vi "imp_test_v1_tmp.vi"() -> ()   [LabVIEW 2014]
uses:
  <vilib>/LabVIEW Targets/FPGA/cRIO/shared/nicrio_ModuleControls/nicrio_cRIO-9237_DataRatesRing.ctl
  <vilib>/LabVIEW Targets/FPGA/cRIO/shared/nicrio_ModuleControls/nicrio_cRIO-9237_ExcitationVoltageRing.ctl
  <vilib>/rvi/FXPMathLib/FxpSinAndCos/subVIs/nifxpmath_SinAndCos_SimConfig.ctl
  <vilib>/Platform/TimedLoop/XDataNode/timing_clust.ctl
  <vilib>/Platform/TimedLoop/XDataNode/nitl_modes.ctl
  <vilib>/Platform/TimedLoop/XDataNode/wakeup.ctl
  <vilib>/rvi/FXPMathLib/basic elements/FxpIntAccumulator/subVIs/nifxpmath_IntAccumulator_SimConfig.ctl
  <vilib>/rvi/FXPMathLib/FxpSqrt/subVIs/nifxpmath_Sqrt_SimConfig.ctl
  <vilib>/fxp/LVFixedPointOverflowPolicyTypeDef.ctl
  <vilib>/rvi/Emulation/niFpgaGetClockAttributes.vi
  <vilib>/rvi/Emulation/niFpgaSctlEmulationGetInTimedLoop.vi
  <vilib>/rvi/Emulation/niFpgaEmulationReportErrorSimple.vi
  <vilib>/rvi/Emulation/niFpgaProcessEmulError.vi
  <vilib>/rvi/interface/RandomDataEmulation/nirviRandomDataMultiElementFPGAFIFO.vi
  <instcachedir>/0/nirviRandomDataMultiElementFPGAFIFO_AD0CFC12EF974623A9C2E4184BC062B2.lvgen/nirviRandomDataMultiElementFPGAFIFO_AD0CFC12EF974623A9C2E4184BC062B2_023.vi
  <vilib>/rvi/interface/RandomDataEmulation/niFpgaRandomDataHandleErrors.vi
  <vilib>/rvi/Emulation/niFpgaCriticalErrorInLSC.vi
  <vilib>/rvi/eio/common/nirviEmuTemplateMethod_errors.vi
  <vilib>/rvi/FXPMathLib/FxpSinAndCos/simVIs/DllFxpSinAndCosTemp_sub.vi
  <vilib>/rvi/eio/common/nirviEmuTemplatePropertySet_errors.vi
  <vilib>/rvi/Analysis/common/codeGenErrors/XNode/niFpgaXNodeCodeGenErrorHandle.vi
  <vilib>/rvi/FXPMathLib/basic elements/FxpIntAccumulator/simVIs/DllFxpIntAccumulator_sub.vi
  <vilib>/rvi/FXPMathLib/FxpSqrt/simVIs/DllSqrtTemp_sub.vi
  <vilib>/rvi/DataTransferAndStorage/Container/XNode/niFpgaContainer.xnode
  <vilib>/rvi/interface/RandomDataEmulation/nirviRandomDataFpgaMultiElementTemplate.vi
  <vilib>/eio/EIONode/EIONode.xnode
  <vilib>/rvi/FXPMathLib/FxpMul/XNode/nifxpmath_Multiplier.xnode
  <vilib>/rvi/FXPMathLib/FxpSinAndCos/XNode/nifxpmath_SinAndCos.xnode
  <vilib>/rvi/Analysis/measure/butterworth/XNode/niFpgaButterworthFilter.xnode
  <vilib>/rvi/FXPMathLib/FxpSub/XNode/nifxpmath_Sub.xnode
  <vilib>/rvi/FXPMathLib/FxpAdd/XNode/nifxpmath_Add.xnode
  <vilib>/eio/EIOPropertyNode/EIOPropertyNode.xnode
  <vilib>/rvi/Analysis/measure/dc-rms/XNode/niFpgaDC-RMS.xnode
  <vilib>/Platform/TimedLoop/XDataNode/XDataNode.xnode
  <vilib>/rvi/FXPMathLib/basic elements/FxpIntAccumulator/XNode/nifxpmath_IntAccumulator.xnode
  <vilib>/rvi/FXPMathLib/FxpSqrt/XNode/nifxpmath_Sqrt.xnode
  <vilib>/rvi/eio/common/nirviEmuTemplatePropertyGet_errors.vi
  <vilib>/rvi/eio/common/nirviEmuTemplatePropertyGet_noerrors.vi
  <vilib>/rvi/eio/common/nirviEmuTemplatePropertySet_noerrors.vi
  <vilib>/Platform/TimedLoop/XDataNode/XDNodeRunTimeDep.lvlib
  <vilib>/rvi/FXPMathLib/sim/FxpSim.dll
panel:
  out "vb":fxp<+/-,38,8>
  out "va":fxp<+/-,38,8>
  out "ft_d2":fxp<+/-,64,59>
  out "Force_r":fxp<+/-,64,42>
  in  "Bv":fxp<+/-,22,8>
  out "D_error_dd":fxp<+/-,64,49>
  out "D_error_d":fxp<+/-,33,10>
  in  "Kv":fxp<+/-,22,8>
  out "D_error":fxp<+/-,64,33>
  out "Dr_sin_dd":fxp<+/-,64,48>
  out "Dr_sin_d":fxp<+/-,64,17>
  out "Sin omega":fxp<+/-,52,9>
  out "Dr_sin":fxp<+/-,39,10>
  in  "Sin offset":fxp<+/-,38,9>
  in  "Sin magnitude":fxp<+/-,22,7>
  out "Time now(s)":fxp<+,52,14>
  in  "Sin wave freq. (Hz)":fxp<+/-,32,6>
  in  "Dr":fxp<+/-,22,7>
  in  "Drive mode":i16(ring) items=["Backward", "Forward"]
  in  "F_d coeff.":i32[](array[numeric])=[946630756, 63555534]
  out "ft_d":fxp<+/-,36,25>
  out "D_dd":fxp<+/-,36,24>
  in  "D_dd coeff.":i32[](array[numeric])=[946630756, 63555534]
  out "dF_PID":fxp<+/-,36,33>
  in  "dF_PID coeff.":i32[](array[numeric])=[946630756, 63555534]
  out "ft_i":fxp<+/-,34,18>
  out "F_PID":fxp<+/-,51,14>
  in  "f_tolorance":fxp<+,22,6>
  in  "Ki":fxp<+/-,36,9>
  in  "Kd":fxp<+/-,36,9>
  out "f_tilde":fxp<+/-,33,11>
  in  "Kp":fxp<+/-,36,9>
  out "vq_F":fxp<+/-,20,5> format="%.57g"
  out "vd_F":fxp<+/-,20,5>
  in  "dF_add":bool
  out "D_d(mm/s)":fxp<+/-,41,10>
  out "omega(rad/s)":fxp<+/-,20,9>
  in  "Veolcity Estimation":i16(ring) items=["T method", "M_avg method", "M method"]
  in  "Stop motor":bool
  out "D_d(T)":fxp<+/-,41,10>
  out "omega(T)":fxp<+/-,20,9>
  in  "mt0_omega":u32
  out "mt_omega":u32
  out "rad(NrTheta)":fxp<+/-,33,10>
  out "D(mm)":fxp<+/-,32,10>
  out "Encoder Position":i32
  in  "Encoder reset":bool
  in  "Ini coe.":bool
  out "Loop rate (kHz)":fxp<+/-,36,7>
  out "Strain (RMS)":fxp<+,32,44>
  in  "Strain filter coeff.":i32[](array[numeric])=[-850883994, 1909449570, 3794062, -975456236, 2033039520, 4039635]
  out "Force":fxp<+/-,32,10>
  out "Strain":fxp<+/-,42,8>
  out "Fileterd data":fxp<+/-,32,4>
  out "Raw Force":fxp<+/-,32,10>
  in  "S/F coeff":fxp<+/-,41,4>
  out "Raw Strain":fxp<+/-,42,8>
  in  "Reset":bool
  in  "Stop (Strain)":bool
  out "Mod6/AI2":fxp<+/-,32,4>
  in  "Shunt Cal Enable":bool
  in  "Half-Bridge Enable":bool
  in  "Excitation Voltage":T1 items=["2.5 Volts", "3.3 Volts", "5.0 Volts", "10.0 Volts", "External Excitation"]
  in  "Data Rate":T2=1 items=["50.000 kS/s (NI 9237)"=1, "25.000 kS/s (NI 9237)"=2, "16.667 kS/s (NI 9237)"=3, "12.500 kS/s (NI 9237)"=4, "10.000 kS/s (NI 9237)"=5, "8.333 kS/s (NI 9237)"=6, "7.143 kS/s (NI 9237)"=7, "6.250 kS/s (NI 9237)"=8, "5.556 kS/s (NI 9237)"=9, "5.000 kS/s (NI 9237)"=10, "4.545 kS/s (NI 9237)"=11, "4.167 kS/s (NI 9237)"=12, "3.846 kS/s (NI 9237)"=13, "3.571 kS/s (NI 9237)"=14, "3.333 kS/s (NI 9237)"=15, "3.125 kS/s (NI 9237)"=16, "2.941 kS/s (NI 9237)"=17, "2.778 kS/s (NI 9237)"=18, "2.632 kS/s (NI 9237)"=19, "2.500 kS/s (NI 9237)"=20, "2.381 kS/s (NI 9237)"=21, "2.273 kS/s (NI 9237)"=22, "2.174 kS/s (NI 9237)"=23, "2.083 kS/s (NI 9237)"=24, "2.000 kS/s (NI 9237)"=25, "1.923 kS/s (NI 9237)"=26, "1.852 kS/s (NI 9237)"=27, "1.786 kS/s (NI 9237)"=28, "1.724 kS/s (NI 9237)"=29, "1.667 kS/s (NI 9237)"=30, "1.613 kS/s (NI 9237)"=31]
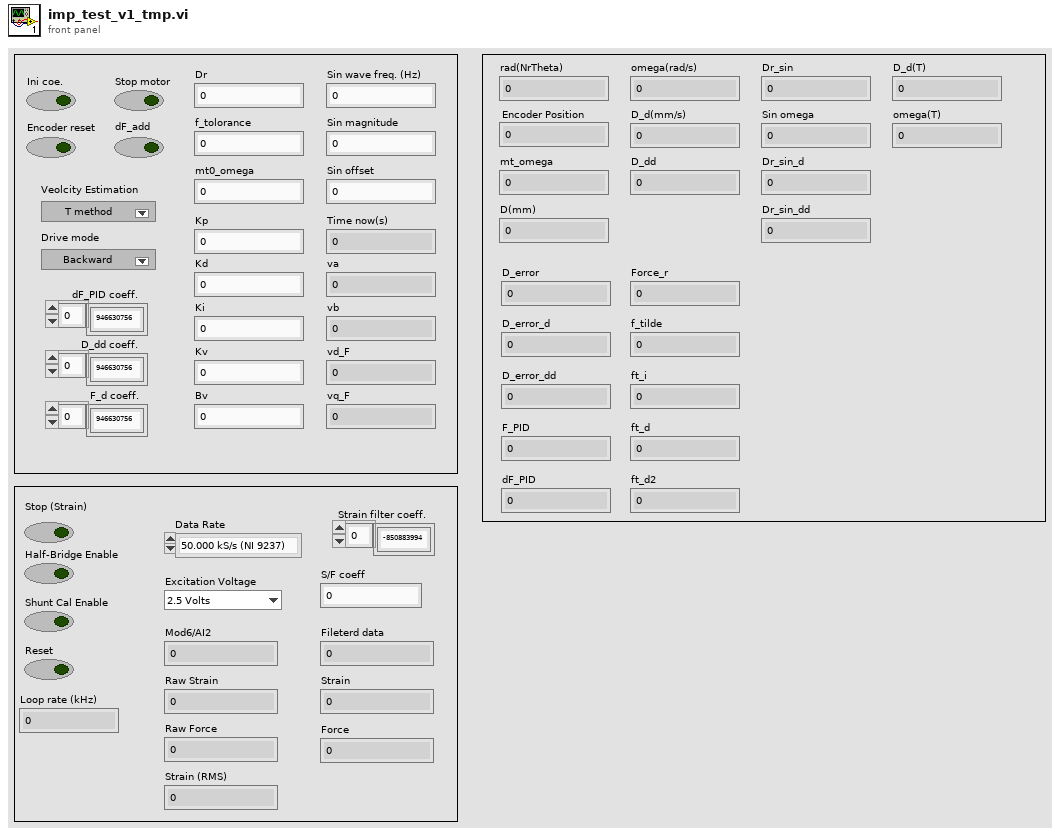
[diagram p1: front panel]
types:
  T1 = typedef "nicrio_cRIO-9237_ExcitationVoltageRing.ctl" = u8
  T2 = typedef "nicrio_cRIO-9237_DataRatesRing.ctl" = u8
  T3 = typedef "XDNodeRunTimeDep.lvlib/timing_clust.ctl" = cluster{"Expected End [f-1]":u64, "Actual End [f-1]":u64, "Finished Late? [f-1]":bool, "Expected End [i-1]":u64, "Actual End [i-1]":u64, "Finished Late? [i-1]":bool, "Expected Start [i]":u64, "Actual Start [i]":u64, "Expected Start [f]":u64, "Actual Start [f]":u64, "Source Name":string, "Structure Name":string, "Period":i64, "Deadline":i64, "Offset":i64, "Start":i64, "Priority":i32, "Timeout":i32, "Mode":T4, "Wakeup Reason":T5, "Error":errorcluster, "Source Type":string, "Secondary Source Type":string, "Global End Time":u64, "Global Start Time":u64, "Frame Duration":u64, "Iteration Duration":u64, "Assigned CPU":i32, "I/O Scan Engine Mode":u32}
  T4 = typedef "XDNodeRunTimeDep.lvlib/nitl_modes.ctl" = enum32{"No Change", "Process missed periods, maintain original phase", "Discard missed periods, maintain original phase", "Process missed periods, ignore original phase", "Discard missed periods, ignore original phase"}
  T5 = typedef "XDNodeRunTimeDep.lvlib/wakeup.ctl" = enum32{"Normal", "Aborted", "Asynchronous wakeup", "Timing source error", "Timed loop error", "Timeout"}
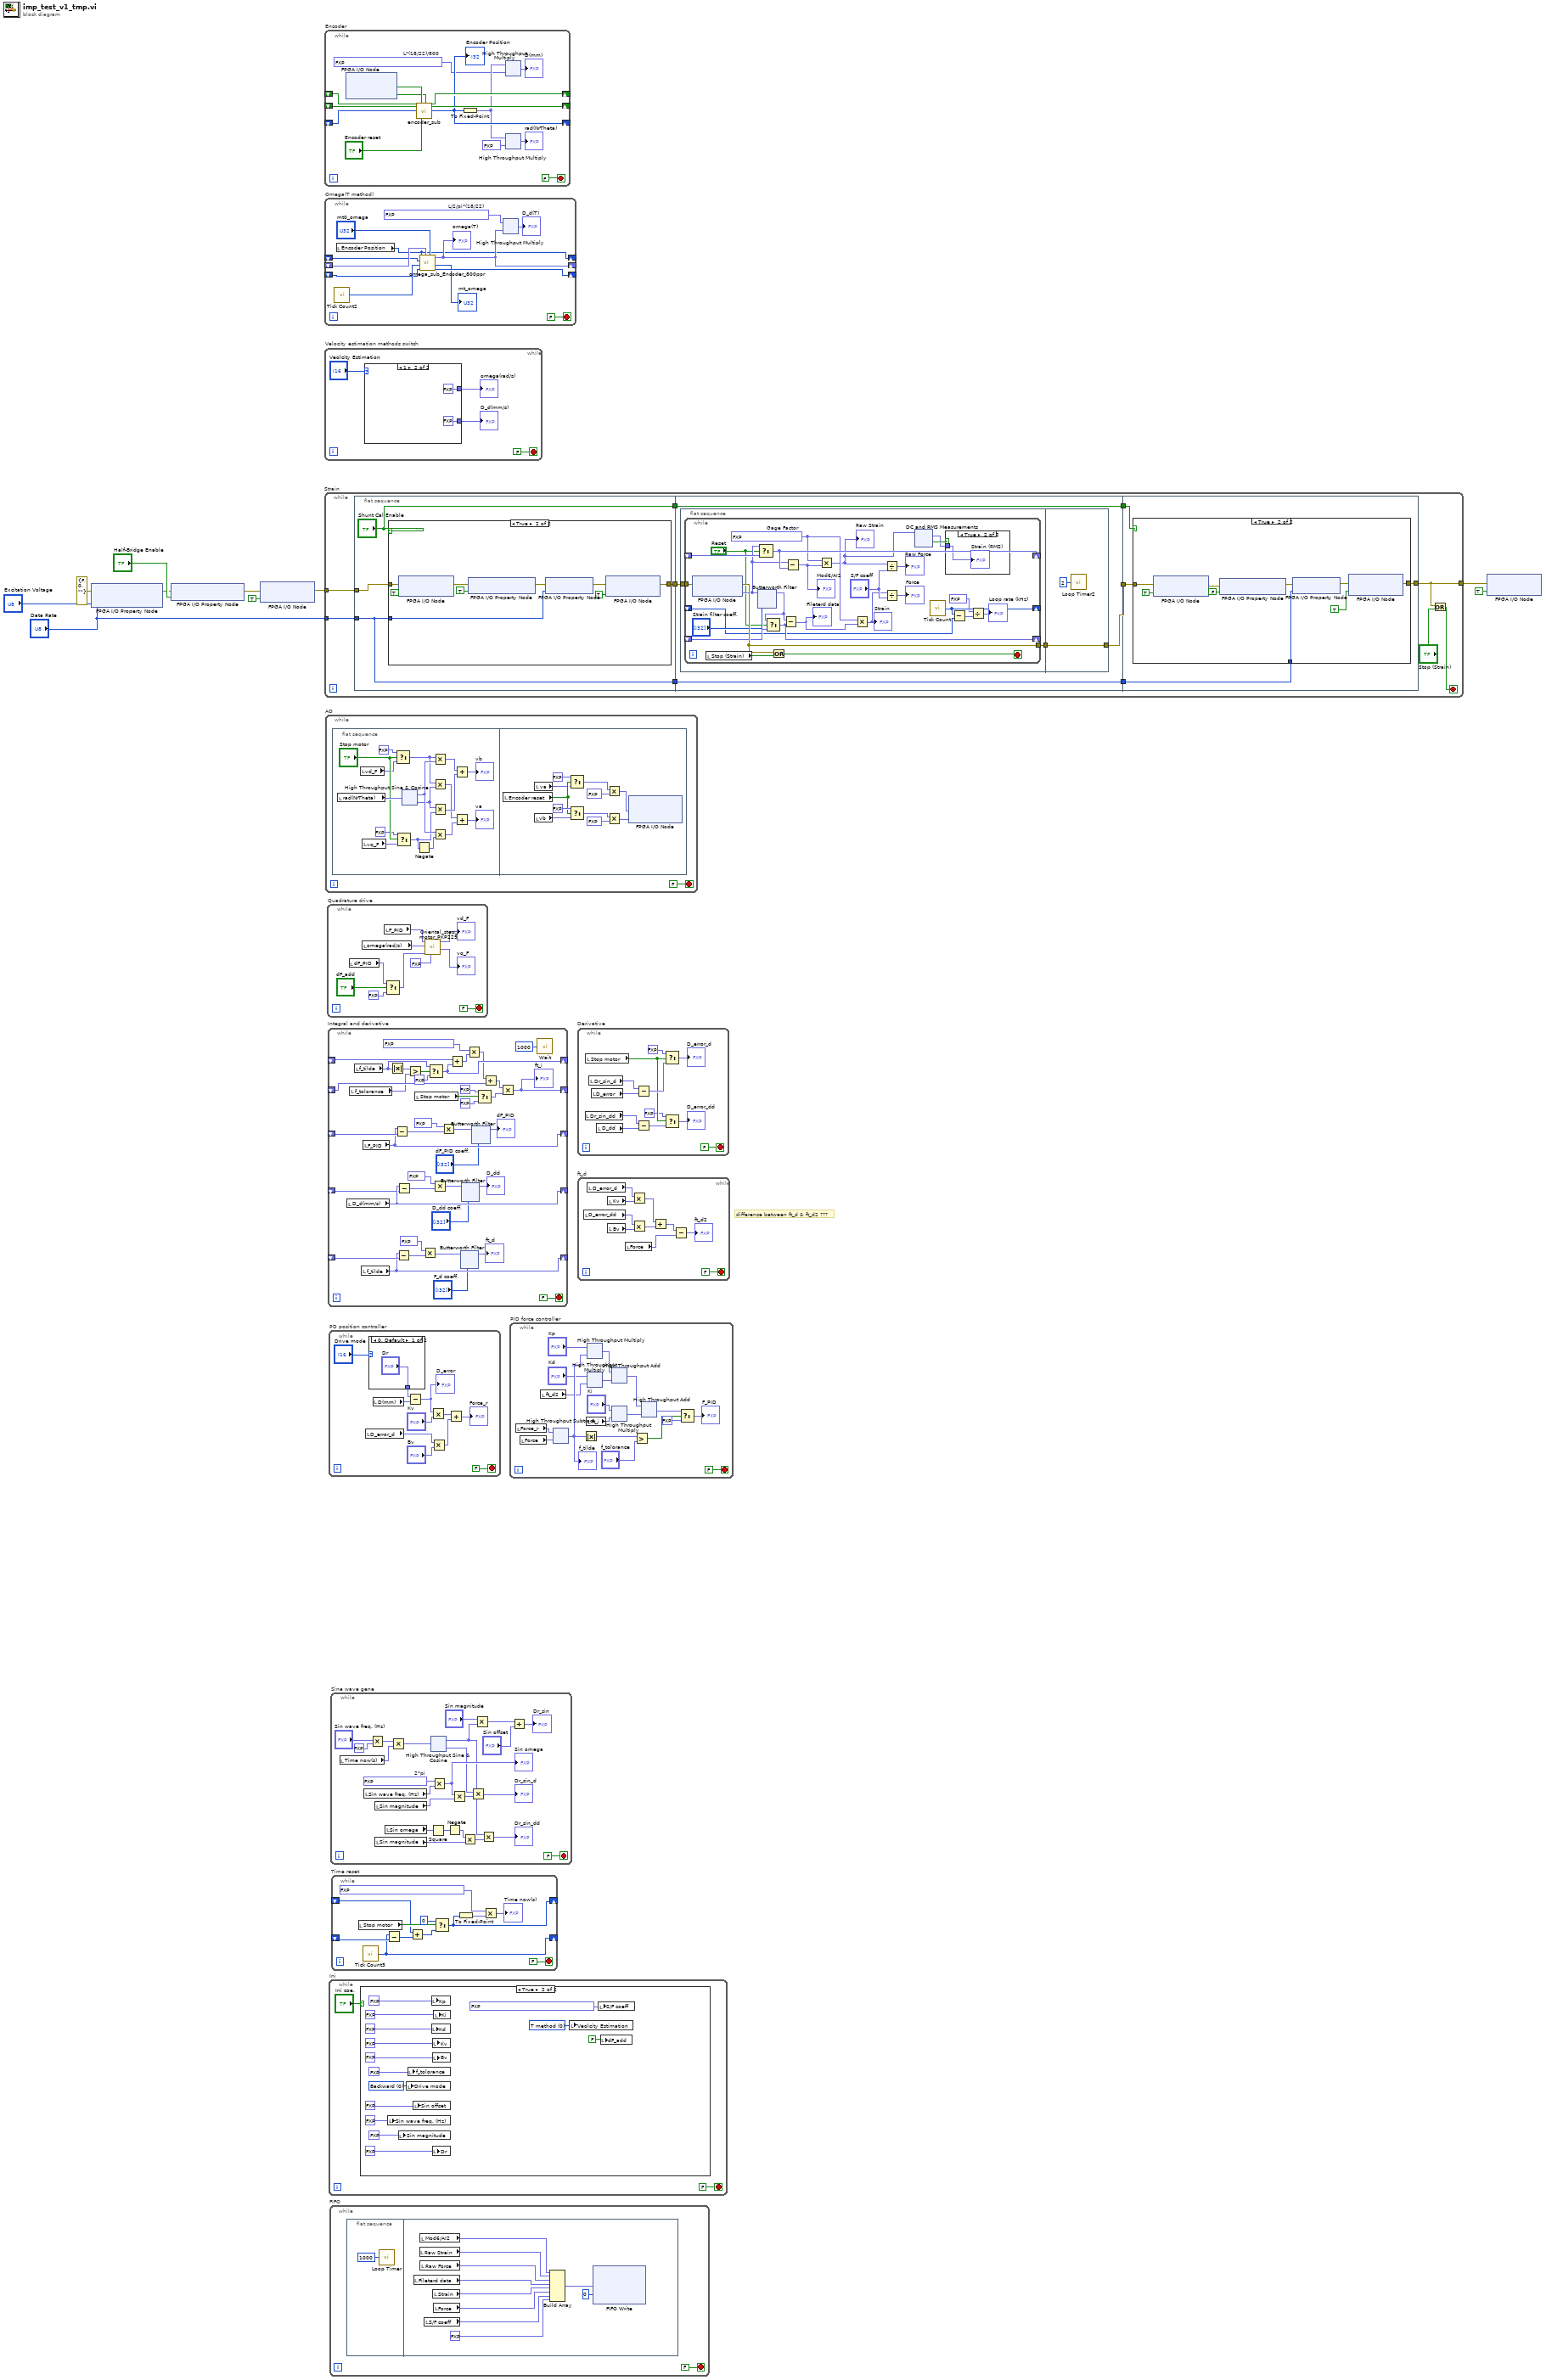
[diagram p0: block diagram]
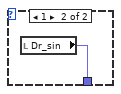
[diagram p2: hidden frame]
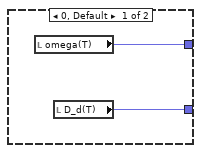
[diagram p3: hidden frame]
diagram:
  # "difference between ft_d & ft_d2 ???"
  n1 = xnode "FPGA I/O Property Node"("error in"=errorcluster {"status"=FALSE, "code"=0, "source"=""}, "Data Rate"="Data Rate", "Excitation Voltage"="Excitation Voltage") -> ("error out"=w7:errorcluster)  [unwired: 1 in, 1 out]
  n2 = xnode "FPGA I/O Property Node"("error in"=w7, "Half-Bridge Enable"="Half-Bridge Enable") -> ("error out"=w6:errorcluster)  [unwired: 1 in, 1 out]
  n3 = xnode "FPGA I/O Node"("error in"=w6, "Mod6/Start"=TRUE) -> ("error out"=w4:errorcluster)  [unwired: 1 in, 1 out]
  n4 = while "Strain" {
    tunnel: w4 -> [w21]
    tunnel: "Data Rate" -> [w20]
    tunnel: [w12] -> w2
    stop <- w13 stop-if-true
    n5 = flat-sequence {
      tunnel: w21 -> [w25]
      tunnel: w20 -> [w24]
      tunnel: [w24] -> w19
      tunnel: ["Shunt Cal Enable"] -> w18
      tunnel: [w22] -> w17
      tunnel: w19 -> [w38]
      tunnel: w18 -> [w39]
      tunnel: w17 -> [w40]
      tunnel: [w39] -> w16
      tunnel: [w37] -> w15
      tunnel: [w38] -> w14
      tunnel: w16 -> [w221]
      tunnel: w15 -> [w220]
      tunnel: w14 -> [w219]
      tunnel: [w218] -> w12
      frame #0 {
        n6 = case shown="True" "Shunt Cal Enable" {
          tunnel: w25 -> [w26 w33]
          tunnel: w24 -> [_ w31]
          tunnel: [w26 w28] -> w22
          frame False {
          }
          frame True {
            n7 = xnode "FPGA I/O Node"("error in"=w33, "Mod6/Stop"=TRUE) -> ("error out"=w34:errorcluster)  [unwired: 1 in, 1 out]
            n8 = xnode "FPGA I/O Property Node"("error in"=w34, "Shunt Cal Enable"=TRUE) -> ("error out"=w32:errorcluster)  [unwired: 1 in, 1 out]
            n9 = xnode "FPGA I/O Property Node"("error in"=w32, "Data Rate"=w31) -> ("error out"=w30:errorcluster)  [unwired: 1 in, 1 out]
            n10 = xnode "FPGA I/O Node"("error in"=w30, "Mod6/Start"=TRUE) -> ("error out"=w28:errorcluster)  [unwired: 1 in, 1 out]
          }
        }
      }
      frame #1 {
        n11 = flat-sequence {
          tunnel: w40 -> [w42]
          tunnel: [w41] -> w36
          tunnel: [w217] -> w37
          tunnel: w36 -> [w217]
          frame #0 {
            n12 = while {
              tunnel: w42 -> [w69]
              tunnel: [w67] -> w41
              shift-right: [w65] -> _
              shift-left: _ -> [w66]
              shift-right: [w61] -> _
              shift-left: _ -> [w62]
              shift-right: [w48] -> _
              shift-left: _ -> [w49]
              stop <- w54 stop-if-true
              w59 = fxp<+,20,2> 2.115001678466797  # Gage Factor
              n13 = xnode "FPGA I/O Node"("error in"=w69) -> ("error out"=w67:errorcluster, "Mod6/AI2"=w63:fxp<+/-,24,-4>)  [unwired: 1 in, 1 out]
              n14 = local read "Stop (Strain)"() -> (w68:bool)
              n15 = xnode "Butterworth Filter"("input data"=w63, "scaled coefficients"="Strain filter coeff.") -> ("output data"=w60:fxp<+/-,28,0>)  [unwired: 1 in]
              n16 = Select(t=w63, s="Reset", f=w66) -> (s? t:f=w65:fxp<+/-,24,-4>)
              n17 = Select(t=w60, s="Reset", f=w62) -> (s? t:f=w61:fxp<+/-,28,0>)
              n18 = Or(x=w67, y=w68) -> (x .or. y?=w54:bool)
              n19 = Subtract(x=w60, y=w61) -> (x-y=w58:fxp<+/-,32,16>)
              "Fileterd data" <- w58
              n20 = Subtract(x=w63, y=w65) -> (x-y=w64:fxp<+/-,25,-3>)
              "Mod6/AI2" <- w64
              n21 = Multiply(x=w59, y=w64) -> (x*y=w46:fxp<+/-,41,6>)
              "Raw Strain" <- w46
              n22 = Multiply(x=w59, y=w58) -> (x*y=w56:fxp<+/-,41,6>)
              "Strain" <- w56
              n23 = Divide(x=w46, y="S/F coeff") -> (x/y=→"Raw Force":fxp<+/-,64,44>)
              n24 = Divide(x=w56, y="S/F coeff") -> (x/y=→"Force":fxp<+/-,64,44>)
              n25 = xnode ("DC and RMS Measurements")("input data"=w46) -> ("RMS"=w50:fxp<+,32,6>, "output valid"=w51:bool)  [unwired: 1 in, 1 out]
              n26 = call "Tick Count"() -> ("Tick Count(uSec)"=w48:u32)
              n27 = case shown="True" w51 {
                tunnel: w50 -> [_ w70]
                frame False {
                }
                frame True {
                  "Strain (RMS)" <- w70
                }
              }
              n28 = Subtract(x=w48, y=w49) -> (x-y=w45:fxp<+/-,32,16>)
              n29 = Divide(x=fxp<+,7,10> 1000.0, y=w45) -> (x/y=→"Loop rate (kHz)":fxp<+/-,40,27>)
            }
          }
          frame #1 {
            n30 = call "Loop Timer2"("Count(uSec)"=u32 2) -> ()  [unwired: 1 out]
          }
        }
      }
      frame #2 {
        n31 = case shown="True" w221 {
          tunnel: w220 -> [w222 w230]
          tunnel: w219 -> [_ w226]
          tunnel: [w222 w223] -> w218
          frame False {
          }
          frame True {
            n32 = xnode "FPGA I/O Node"("error in"=w230, "Mod6/Stop"=TRUE) -> ("error out"=w228:errorcluster)  [unwired: 1 in, 1 out]
            n33 = xnode "FPGA I/O Property Node"("error in"=w228, "Shunt Cal Enable"=FALSE) -> ("error out"=w227:errorcluster)  [unwired: 1 in, 1 out]
            n34 = xnode "FPGA I/O Property Node"("error in"=w227, "Data Rate"=w226) -> ("error out"=w225:errorcluster)  [unwired: 1 in, 1 out]
            n35 = xnode "FPGA I/O Node"("error in"=w225, "Mod6/Start"=TRUE) -> ("error out"=w223:errorcluster)  [unwired: 1 in, 1 out]
          }
        }
      }
    }
    n36 = Or(x=w12, y="Stop (Strain)") -> (x .or. y?=w13:bool)
  }
  n37 = while "Encoder" {
    shift-right: [w243] -> _
    shift-left: _ -> [w244]
    shift-right: [w245] -> _
    shift-left: _ -> [w246]
    shift-right: [w238] -> _
    shift-left: _ -> [w242]
    stop <- FALSE stop-if-true
    w235 = fxp<+/-,32,0> 0.0020454544574022293  # L*(18/22)/800
    n38 = xnode "FPGA I/O Node"() -> ("Mod4/DI3"=w241:bool, "Mod4/DI4"=w240:bool)  [unwired: 2 in, 2 out]
    n39 = call "encoder_sub.vi"("A_pre"=w244, "B_pre"=w246, "Encoder Position_pre"=w242, "A input"=w241, "Encoder Position Reset"="Encoder reset", "B input"=w240) -> ("A"=w243:bool, "B"=w245:bool, "Encoder Position (Counts)"=w238:i32)  [unwired: 19 in]
    "Encoder Position" <- w238
    n40 = To Fixed-Point(number=w238) -> (fixed-point=w237:fxp<+/-,32,32>)  [unwired: 1 in]
    n41 = xnode "High Throughput Multiply"("x"=w237, "y"=w235) -> ("x*y"=→"D(mm)":fxp<+/-,64,32>)
    n42 = xnode "High Throughput Multiply"("x"=w237, "y"=fxp<+/-,16,1> 0.125) -> ("x*y"=→"rad(NrTheta)":fxp<+/-,48,33>)
  }
  n43 = while "Omega(T method)" {
    shift-right: [w248] -> _
    shift-left: _ -> [w249]
    shift-right: [w252] -> _
    shift-left: _ -> [w254]
    shift-right: [w256] -> _
    shift-left: _ -> [w257]
    stop <- FALSE stop-if-true
    w251 = fxp<+/-,32,0> 0.2604353614151478  # L/2/pi*(18/22)
    n44 = call "Tick Count2"() -> ("Tick Count(Ticks)"=w258:u32)
    n45 = local read "Encoder Position"() -> (w248:i32)
    n46 = call "omega_sub_Encoder_800ppr.vi"("mt0"="mt0_omega", "omega_pre"=w254, "ticks_m_pre"=w257, "ticks"=w258, "count_pre"=w249, "count"=w248) -> ("ticks_m"=w256:u32, "mt"=→"mt_omega":u32, "omega"=w252:fxp<+/-,20,9>)  [unwired: 3 in]
    "omega(T)" <- w252
    n47 = xnode "High Throughput Multiply"("x"=w251, "y"=w252) -> ("x*y"=→"D_d(T)":fxp<+/-,52,9>)
  }
  n48 = while "Velocity estimation methods switch" {
    stop <- FALSE stop-if-true
    n49 = case shown="1" "Veolcity Estimation" {
      tunnel: [w264 fxp<+/-,20,9> 0.0 ("omega(T)")] -> w261
      tunnel: [w263 fxp<+/-,41,10> 0.0 ("D_d(T)")] -> w260
      frame 0, Default {
        n50 = local read "omega(T)"() -> (w264:fxp<+/-,20,9>)
        n51 = local read "D_d(T)"() -> (w263:fxp<+/-,41,10>)
      }
      frame 1 {
      }
    }
    "omega(rad/s)" <- w261
    "D_d(mm/s)" <- w260
  }
  n52 = while "AO" {
    stop <- FALSE stop-if-true
    n53 = flat-sequence {
      frame #0 {
        n54 = local read "rad(NrTheta)"() -> (w284:fxp<+/-,33,10>)
        n55 = local read "vd_F"() -> (w282:fxp<+/-,20,5>)
        n56 = local read "vq_F"() -> (w281:fxp<+/-,20,5>)
        n57 = Select(t=fxp<+/-,20,5> 0.0, s="Stop motor", f=w282) -> (s? t:f=w276:fxp<+/-,20,5>)
        n58 = Select(t=fxp<+/-,20,5> 0.0, s="Stop motor", f=w281) -> (s? t:f=w275:fxp<+/-,20,5>)
        n59 = xnode "High Throughput Sine & Cosine"("x (pi)"=w284) -> ("sin(x)"=w278:fxp<+/-,17,2>, "cos(x)"=w277:fxp<+/-,17,2>)
        n60 = Negate(x=w275) -> (-x=w274:fxp<+/-,21,6>)
        n61 = Multiply(x=w276, y=w278) -> (x*y=w273:fxp<+/-,37,7>)
        n62 = Multiply(x=w276, y=w277) -> (x*y=w271:fxp<+/-,37,7>)
        n63 = Multiply(x=w277, y=w275) -> (x*y=w272:fxp<+/-,37,7>)
        n64 = Multiply(x=w278, y=w274) -> (x*y=w270:fxp<+/-,36,6>)
        n65 = Add(x=w273, y=w272) -> (x+y=→"vb":fxp<+/-,38,8>)
        n66 = Add(x=w271, y=w270) -> (x+y=→"va":fxp<+/-,37,7>)
      }
      frame #1 {
        n67 = local read "Encoder reset"() -> (w317:bool)
        n68 = local read "vb"() -> (w315:fxp<+/-,38,8>)
        n69 = local read "va"() -> (w316:fxp<+/-,38,8>)
        n70 = Select(t=fxp<+,2,2> 3.0, s=w317, f=w316) -> (s? t:f=w321:fxp<+/-,38,8>)
        n71 = Select(t=fxp<+,1,1> 0.0, s=w317, f=w315) -> (s? t:f=w320:fxp<+/-,38,8>)
        n72 = Multiply(x=w321, y=fxp<+/-,1,0> -0.5) -> (x*y=w324:fxp<+/-,39,8>)
        n73 = Multiply(x=w320, y=fxp<+/-,1,0> -0.5) -> (x*y=w325:fxp<+/-,37,6>)
        n74 = xnode "FPGA I/O Node"("Mod8/AO2"=w324, "Mod8/AO3"=w325) -> ()  [unwired: 2 in, 2 out]
      }
    }
  }
  n75 = while "Quadrature drive" {
    stop <- FALSE stop-if-true
    n76 = local read "dF_PID"() -> (w327:fxp<+/-,36,33>)
    n77 = local read "omega(rad/s)"() -> (w335:fxp<+/-,20,9>)
    n78 = local read "F_PID"() -> (w328:fxp<+/-,51,14>)
    n79 = Select(t=w327, s="dF_add", f=fxp<+,1,1> 0.0) -> (s? t:f=w331:fxp<+/-,36,33>)
    n80 = call "Oriental_step_motor_PKP225.vi"("F_Threshold"=fxp<+,12,12> 10.0, "dFmr"=w331, "omega"=w335, "Fmr"=w328) -> ("vq_F"=→"vq_F":fxp<+/-,20,5>, "vd_F"=→"vd_F":fxp<+/-,20,5>)  [unwired: 6 in]
  }
  n81 = while "Integral and derivative" {
    shift-right: [w367] -> _
    shift-left: _ -> [w366]
    shift-right: [w359] -> _
    shift-left: _ -> [w358]
    shift-right: [w369] -> _
    shift-left: _ -> [w370]
    shift-right: [w349] -> _
    shift-left: _ -> [w348]
    shift-right: [w341] -> _
    shift-left: _ -> [w345]
    stop <- FALSE stop-if-true
    n82 = local read "D_d(mm/s)"() -> (w349:fxp<+/-,41,10>)
    n83 = local read "f_tolorance"() -> (w336:fxp<+,22,6>)
    n84 = local read "f_tilde"() -> (w371:fxp<+/-,33,11>)
    n85 = local read "f_tilde"() -> (w341:fxp<+/-,33,11>)
    n86 = local read "F_PID"() -> (w369:fxp<+/-,51,14>)
    n87 = Absolute Value(x=w371) -> (abs(x)=w373:fxp<+,33,11>)
    n88 = Subtract(x=w369, y=w370) -> (x-y=w357:fxp<+/-,52,15>)
    n89 = Subtract(x=w341, y=w345) -> (x-y=w344:fxp<+/-,34,12>)
    n90 = Subtract(x=w349, y=w348) -> (x-y=w351:fxp<+/-,42,11>)
    n91 = Greater?(x=w373, y=w336) -> (0:w374:bool)
    n92 = local read "Stop motor"() -> (w360:bool)
    n93 = Multiply(x=fxp<+/-,33,11> 1000.0, y=w344) -> (x*y=w342:fxp<+/-,64,22>)
    n94 = Select(t=w371, s=w374, f=fxp<+/-,33,11> 0.0) -> (s? t:f=w367:fxp<+/-,33,11>)
    n95 = Multiply(x=fxp<+,7,10> 1000.0, y=w351) -> (x*y=w350:fxp<+/-,49,21>)
    n96 = Multiply(x=fxp<+/-,52,15> 1000.0, y=w357) -> (x*y=w354:fxp<+/-,64,29>)
    n97 = Add(x=w366, y=w367) -> (x+y=w372:fxp<+/-,34,12>)
    n98 = xnode "Butterworth Filter"("input data"=w342, "scaled coefficients"="F_d coeff.") -> ("output data"=→"ft_d":fxp<+/-,36,26>)  [unwired: 1 in]
    n99 = xnode "Butterworth Filter"("input data"=w350, "scaled coefficients"="D_dd coeff.") -> ("output data"=→"D_dd":fxp<+/-,36,25>)  [unwired: 1 in]
    n100 = Multiply(x=fxp<+/-,30,12> 0.000499725341796875, y=w372) -> (x*y=w365:fxp<+/-,64,24>)
    n101 = xnode "Butterworth Filter"("input data"=w354, "scaled coefficients"="dF_PID coeff.") -> ("output data"=→"dF_PID":fxp<+/-,36,33>)  [unwired: 1 in]
    n102 = Select(t=fxp<+,1,1> 0.0, s=w360, f=fxp<+,1,1> 1.0) -> (s? t:f=w363:fxp<+,1,1>)
    n103 = Add(x=w365, y=w358) -> (x+y=w364:fxp<+/-,64,24>)
    n104 = Multiply(x=w364, y=w363) -> (x*y=w359:fxp<+/-,34,18>)
    "ft_i" <- w359
    n105 = call "Wait"("Count(uSec)"=u32 1000) -> ()  [unwired: 1 out]
  }
  n106 = while "PD position controller" {
    stop <- FALSE stop-if-true
    n107 = local read "D_error_d"() -> (w403:fxp<+/-,33,10>)
    n108 = case shown="0, Default" "Drive mode" {
      tunnel: ["Dr" w412] -> w408
      frame 0, Default {
      }
      frame 1 {
        n109 = local read "Dr_sin"() -> (w412:fxp<+/-,39,10>)
      }
    }
    n110 = local read "D(mm)"() -> (w409:fxp<+/-,32,10>)
    n111 = Subtract(x=w408, y=w409) -> (x-y=w407:fxp<+/-,40,11>)
    "D_error" <- w407
    n112 = Multiply(x=w407, y="Kv") -> (x*y=w405:fxp<+/-,61,18>)
    n113 = Multiply(x=w403, y="Bv") -> (x*y=w402:fxp<+/-,55,18>)
    n114 = Add(x=w405, y=w402) -> (x+y=→"Force_r":fxp<+/-,62,19>)
  }
  n115 = while "Ini" {
    stop <- FALSE stop-if-true
    n116 = case shown="True" "Ini coe." {
      frame False {
      }
      frame True {
        w420 = i16 0 items=["T method", "M_avg method", "M method"] ("Veolcity Estimation")
        w422 = i16 0 items=["Backward", "Forward"] ("Drive mode")
        n117 = local write "Sin wave freq. (Hz)"(fxp<+/-,32,6> 1.0 ("Sin wave freq. (Hz)")) -> ()
        n118 = local write "Sin magnitude"(fxp<+/-,22,7> 10.0 ("Sin magnitude")) -> ()
        n119 = local write "Drive mode"(w422) -> ()
        n120 = local write "f_tolorance"(fxp<+,22,6> 10.0 ("f_tolorance")) -> ()
        n121 = local write "Sin offset"(fxp<+/-,38,9> 0.0 ("Sin offset")) -> ()
        n122 = local write "Kp"(fxp<+/-,36,9> 50.0 ("Kp")) -> ()
        n123 = local write "Kd"(fxp<+/-,36,9> 0.0 ("Kd")) -> ()
        n124 = local write "Kv"(fxp<+/-,22,8> 1.0 ("Kv")) -> ()
        n125 = local write "Bv"(fxp<+/-,22,8> 0.0 ("Bv")) -> ()
        n126 = local write "Dr"(fxp<+/-,22,7> 0.0 ("Dr")) -> ()
        n127 = local write "Ki"(fxp<+/-,36,9> 0.0 ("Ki")) -> ()
        n128 = local write "Veolcity Estimation"(w420) -> ()
        n129 = local write "S/F coeff"(fxp<+/-,41,4> 1.047803380060941e-06 ("S/F coeff")) -> ()
        n130 = local write "dF_add"(FALSE ("dF_add")) -> ()
      }
    }
  }
  n131 = while "FIFO" {
    stop <- FALSE stop-if-true
    n132 = flat-sequence {
      frame #0 {
        n133 = call "Loop Timer"("Count(uSec)"=u32 1000) -> ()  [unwired: 1 out]
      }
      frame #1 {
        n134 = local read "Fileterd data"() -> (w437:fxp<+/-,32,4>)
        n135 = local read "Raw Strain"() -> (w439:fxp<+/-,42,8>)
        n136 = local read "Mod6/AI2"() -> (w440:fxp<+/-,32,4>)
        n137 = local read "Raw Force"() -> (w438:fxp<+/-,32,10>)
        n138 = local read "S/F coeff"() -> (w434:fxp<+/-,41,4>)
        n139 = local read "Strain"() -> (w436:fxp<+/-,42,8>)
        n140 = local read "Force"() -> (w435:fxp<+/-,32,10>)
        n141 = Build Array(w440, w439, w438, w437, w436, w435, w434, fxp<+,1,1> 0.0) -> (w432:fxp<+/-,47,10>[])
        n142 = xnode ("FIFO Write")("Element"=w432, "Timeout"=0) -> ()  [unwired: 1 in, 2 out]
      }
    }
  }
  n143 = while "Sine wave gene" {
    stop <- FALSE stop-if-true
    w455 = fxp<+,20,3> 6.2831878662109375  # 2*pi
    n144 = local read "Time now(s)"() -> (w461:fxp<+,52,14>)
    n145 = local read "Sin wave freq. (Hz)"() -> (w454:fxp<+/-,32,6>)
    n146 = Multiply(x="Sin wave freq. (Hz)", y=fxp<+/-,32,6> 2.0) -> (x*y=w462:fxp<+/-,64,12>)
    n147 = local read "Sin magnitude"() -> (w452:fxp<+/-,22,7>)
    n148 = local read "Sin magnitude"() -> (w445:fxp<+/-,22,7>)
    n149 = local read "Sin omega"() -> (w448:fxp<+/-,52,9>)
    n150 = Multiply(x=w462, y=w461) -> (x*y=w460:fxp<+/-,64,25>)
    n151 = Square(x=w448) -> (x^2=w447:fxp<+,64,16>)
    n152 = xnode "High Throughput Sine & Cosine"("x (pi)"=w460) -> ("sin(x)"=w442:fxp<+/-,16,2>, "cos(x)"=w450:fxp<+/-,16,2>)
    n153 = Multiply(x=w455, y=w454) -> (x*y=w453:fxp<+/-,52,9>)
    "Sin omega" <- w453
    n154 = Negate(x=w447) -> (-x=w446:fxp<+/-,64,17>)
    n155 = Multiply(x=w453, y=w452) -> (x*y=w451:fxp<+/-,64,15>)
    n156 = Multiply(x=w446, y=w445) -> (x*y=w444:fxp<+/-,64,24>)
    n157 = Multiply(x=w450, y=w451) -> (x*y=→"Dr_sin_d":fxp<+/-,64,17>)
    n158 = Multiply(x="Sin magnitude", y=w442) -> (x*y=w458:fxp<+/-,38,9>)
    n159 = Multiply(x=w442, y=w444) -> (x*y=→"Dr_sin_dd":fxp<+/-,64,26>)
    n160 = Add(x=w458, y="Sin offset") -> (x+y=→"Dr_sin":fxp<+/-,39,10>)
  }
  n161 = while "Time reset" {
    shift-right: [w504] -> _
    shift-left: _ -> [w505]
    shift-right: [w499] -> _
    shift-left: _ -> [w500]
    stop <- FALSE stop-if-true
    n162 = local read "Stop motor"() -> (w506:bool)
    n163 = call "Tick Count3"() -> ("Tick Count(uSec)"=w504:u32)
    n164 = Subtract(x=w504, y=w505) -> (x-y=w503:u32)
    n165 = Add(x=w500, y=w503) -> (x+y=w502:u32)
    n166 = Select(t=u32 0, s=w506, f=w502) -> (s? t:f=w499:u32)
    n167 = To Fixed-Point(number=w499) -> (fixed-point=w498:fxp<+,32,32>)  [unwired: 1 in]
    n168 = Multiply(x=fxp<+,20,-18> 1.0000003385357559e-06, y=w498) -> (x*y=→"Time now(s)":fxp<+,52,14>)
  }
  n169 = while "PID force controller" {
    stop <- FALSE stop-if-true
    n170 = local read "Force_r"() -> (w510:fxp<+/-,64,42>)
    n171 = local read "Force"() -> (w524:fxp<+/-,32,10>)
    n172 = local read "ft_d2"() -> (w509:fxp<+/-,64,59>)
    n173 = xnode "High Throughput Subtract"("x"=w510, "y"=w524) -> ("x-y"=w523:fxp<+/-,64,43>)
    "f_tilde" <- w523
    n174 = Absolute Value(x=w523) -> (abs(x)=w514:fxp<+,64,43>)
    n175 = local read "ft_i"() -> (w508:fxp<+/-,34,18>)
    n176 = xnode "High Throughput Multiply"("x"="Kp", "y"=w523) -> ("x*y"=w521:fxp<+/-,64,52>)
    n177 = xnode "High Throughput Multiply"("x"="Kd", "y"=w509) -> ("x*y"=w520:fxp<+/-,64,68>)
    n178 = xnode "High Throughput Add"("x"=w521, "y"=w520) -> ("x+y"=w517:fxp<+/-,64,69>)
    n179 = xnode "High Throughput Multiply"("x"="Ki", "y"=w508) -> ("x*y"=w518:fxp<+/-,64,27>)
    n180 = Greater?(x=w514, y="f_tolorance") -> (0:w512:bool)
    n181 = xnode "High Throughput Add"("x"=w517, "y"=w518) -> ("x+y"=w516:fxp<+/-,64,70>)
    n182 = Select(t=w516, s=w512, f=fxp<+/-,51,14> 0.0) -> (s? t:f=→"F_PID":fxp<+/-,64,70>)
  }
  n183 = while "Derivative" {
    stop <- FALSE stop-if-true
    n184 = local read "Dr_sin_dd"() -> (w531:fxp<+/-,64,48>)
    n185 = local read "Stop motor"() -> (w529:bool)
    n186 = local read "Dr_sin_d"() -> (w534:fxp<+/-,64,17>)
    n187 = local read "D_error"() -> (w535:fxp<+/-,64,33>)
    n188 = local read "D_dd"() -> (w532:fxp<+/-,36,24>)
    n189 = Subtract(x=w534, y=w535) -> (x-y=w533:fxp<+/-,64,34>)
    n190 = Subtract(x=w531, y=w532) -> (x-y=w530:fxp<+/-,64,49>)
    n191 = Select(t=fxp<+,1,1> 0.0, s=w529, f=w533) -> (s? t:f=→"D_error_d":fxp<+/-,64,34>)
    n192 = Select(t=fxp<+/-,64,49> 0.0, s=w529, f=w530) -> (s? t:f=→"D_error_dd":fxp<+/-,64,49>)
  }
  n193 = while "ft_d" {
    stop <- FALSE stop-if-true
    n194 = local read "D_error_dd"() -> (w544:fxp<+/-,64,49>)
    n195 = local read "D_error_d"() -> (w546:fxp<+/-,33,10>)
    n196 = local read "Kv"() -> (w547:fxp<+/-,22,8>)
    n197 = local read "Bv"() -> (w545:fxp<+/-,22,8>)
    n198 = local read "Force"() -> (w540:fxp<+/-,32,10>)
    n199 = Multiply(x=w546, y=w547) -> (x*y=w542:fxp<+/-,55,18>)
    n200 = Multiply(x=w544, y=w545) -> (x*y=w543:fxp<+/-,64,57>)
    n201 = Add(x=w542, y=w543) -> (x+y=w541:fxp<+/-,64,58>)
    n202 = Subtract(x=w541, y=w540) -> (x-y=→"ft_d2":fxp<+/-,64,59>)
  }
  n203 = xnode "FPGA I/O Node"("error in"=w2, "Mod6/Stop"=TRUE) -> ()  [unwired: 1 in, 2 out]
